vi "Discrete LQR.vi"(9 "R":T1, 10 "Q":T1, 11 "State Space Model":T2) -> (1 "X":T1, 3 "K":T1)   [LabVIEW 2020]
uses:
  State Space/State Space.ctl
  <vilib>/Analysis/Matrix/Datatypes/RealMatrix.ctl
  <vilib>/Analysis/7linalg.llb/Real Transpose Matrix.vi
  <vilib>/Analysis/baseanly.llb/Real A x B.vi
  <vilib>/Analysis/Matrix/Numeric/Add/Add - RM,RM.vi
  <vilib>/Analysis/7linalg.llb/Solve Linear Equations (multiple right hand).vi
  <vilib>/Analysis/NI_AALPro.lvlib
  <vilib>/Analysis/NI_AALBase.lvlib
  <vilib>/Analysis/Matrix/NI_Matrix.lvlib
panel:
  out "x/y":T1
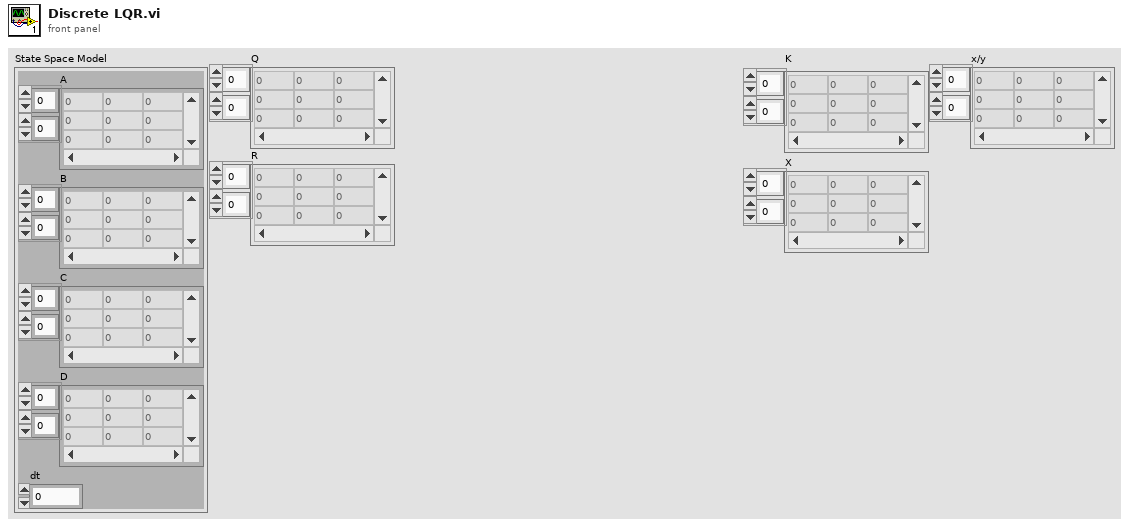
[diagram p1: front panel]
types:
  T1 = typedef "NI_Matrix.lvlib/RealMatrix.ctl" = dbl[][]
  T2 = typedef "State Space.ctl" = cluster{"A":T1, "B":T1, "C":T1, "D":T1, "dt":dbl}
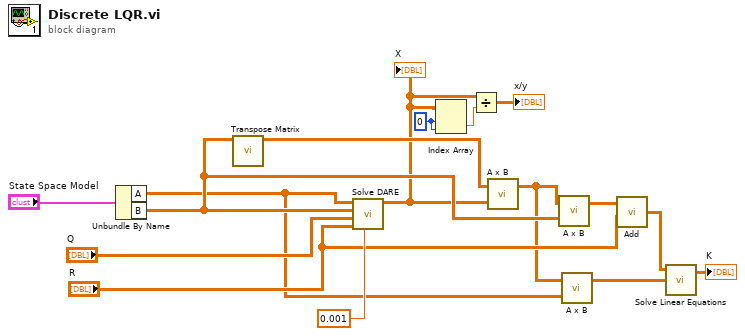
[diagram p0: block diagram]
diagram:
  w3 = 0 ("index (row)")
  n1 = Unbundle By Name("State Space Model") -> ("A"=w8:T1, "B"=w12:T1)
  n2 = call-poly <vilib>:"Transpose Matrix.vi"("Input Matrix"=w12) -> ("Matrix Transpose"=w13:T1)  [unwired: 9 in, 1 out]
  n3 = call "Solve DARE.vi"("epsilon"=0.001, "R"="R", "Q"="Q", "B"=w12, "A"=w8) -> ("X"=w4:T1)  [unwired: 6 in]
  "X" <- w4
  n4 = Index Array(array=w4, index (row)=w3, index (col)=w3) -> (element=w2:dbl)
  n5 = Divide(x=w4, y=w2) -> (x/y=→"x/y":T1)
  n6 = call-poly <vilib>:"A x B.vi"("B"=w4, "A"=w13) -> ("A x B"=w9:T1)  [unwired: 1 out]
  n7 = call-poly <vilib>:"A x B.vi"("B"=w12, "A"=w9) -> ("A x B"=w11:T1)  [unwired: 1 out]
  n8 = call-poly <vilib>:"A x B.vi"("B"=w8, "A"=w9) -> ("A x B"=w7:T1)  [unwired: 1 out]
  n9 = call-poly <vilib>:"Add.vi"("Real Matrix B"="R", "Real Matrix A"=w11) -> ("A + B"=w6:T1)
  n10 = call-poly <vilib>:"Solve Linear Equations.vi"("Known Matrix"=w7, "Input Matrix"=w6) -> ("Solution Matrix"=→"K":T1)  [unwired: 1 in, 1 out]
